vi "Compare_odour_bottles.vi"(9 "Bottle 2":T1, 10 "Bottle 1":T1, 11 "Odour component data":T2) -> (3 "distance":dbl)   [LabVIEW 2016]
uses:
  <vilib>/Analysis/baseanly.llb/Mean (DBL).vi
  <vilib>/Analysis/NI_AALBase.lvlib
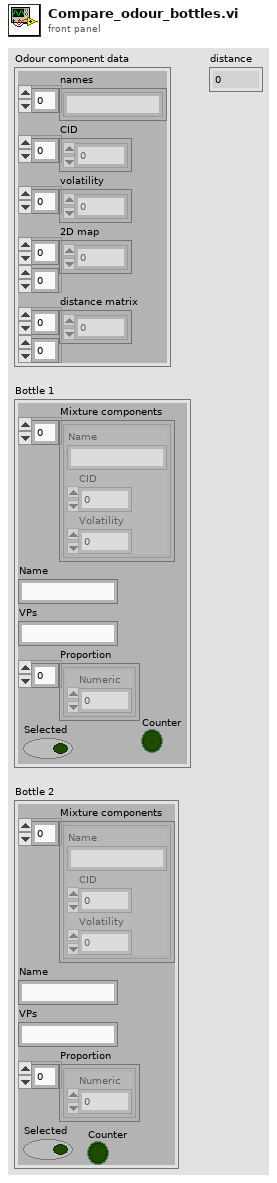
[diagram p1: front panel]
types:
  T1 = cluster{"Mixture components":cluster{"Name":string, "CID":i32, "Volatility":dbl}[], "Name":string, "VPs":string, "Proportion":cluster{"Numeric":dbl}[], "Selected":bool, "Counter":bool}
  T2 = cluster{"names":string[], "CID":i32[], "volatility":dbl[], "2D map":dbl[][], "distance matrix":dbl[][]}
  T3 = cluster{"Name":string, "CID":i32, "Volatility":dbl}[]
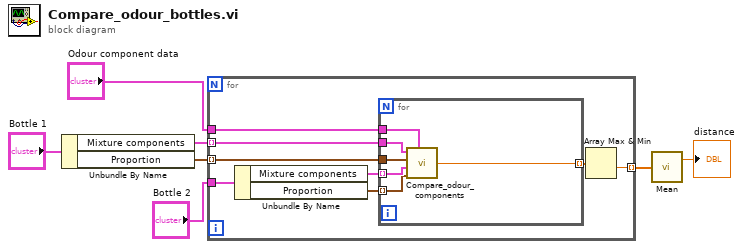
[diagram p0: block diagram]
diagram:
  n1 = Unbundle By Name("Bottle 1") -> ("Mixture components"=w6:T3, "Proportion"=w4:cluster{"Numeric":dbl}[])
  n2 = for {
    tunnel: w6 -> [w14] mode=indexing
    tunnel: "Bottle 2" -> [w15]
    tunnel: w4 -> [w13] mode=indexing
    tunnel: "Odour component data" -> [w10]
    tunnel: [w8] -> w1 mode=indexing
    n3 = Unbundle By Name(w15) -> ("Mixture components"=w11:T3, "Proportion"=w12:cluster{"Numeric":dbl}[])
    n4 = for {
      tunnel: w14 -> [w20]
      tunnel: w11 -> [w18] mode=indexing
      tunnel: w13 -> [w19]
      tunnel: w12 -> [w17] mode=indexing
      tunnel: [w21] -> w9 mode=indexing
      tunnel: w10 -> [w16]
      n5 = call "Compare_odour_components.vi"("Odour component 1"=w20, "Proportion 1"=w19, "Odour component 2"=w18, "Proportion 2"=w17, "Odour component data"=w16) -> ("Distance"=w21:dbl)  [unwired: 2 in]
    }
    n6 = Array Max & Min(array=w9) -> (min value=w8:dbl)  [unwired: 3 out]
  }
  n7 = call-poly <vilib>:"Mean.vi"("X"=w1) -> ("mean"=→"distance":dbl)  [unwired: 1 out]
